vi "Configure RawData.vi"(7 "status?":bool, 8 "error in":errorcluster caption="error in (no error)", 9 "option":i32(ring) items=["ELEM", "SAVE"], 10 "channel":i32(ring) items=["ELEM1", "ELEM2", "ELEM3", "ELEM4", "ELEM5", "ELEM6", "ELEM7"], 11 "VISA resource name":refnum<visa-resource-name>) -> (0 "error out":errorcluster, 3 "VISA resource out":refnum<visa-resource-name>)   [LabVIEW 2018, in "Suita SPAW7000.lvlib"]
uses:
  <instrlib>/Suita SPAW7000/Suita SPAW7000.lvlib
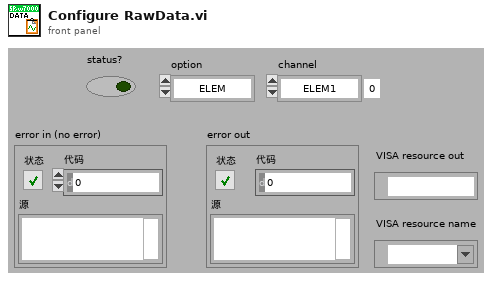
[diagram p1: front panel]
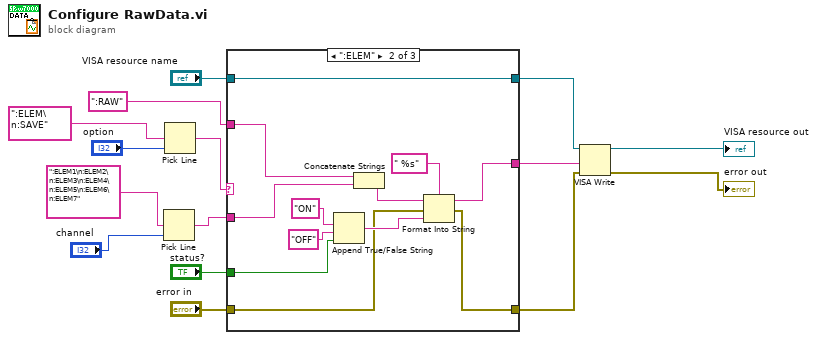
[diagram p0: block diagram]
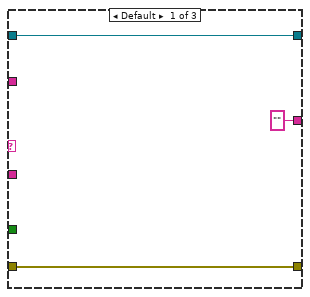
[diagram p2: hidden frame]
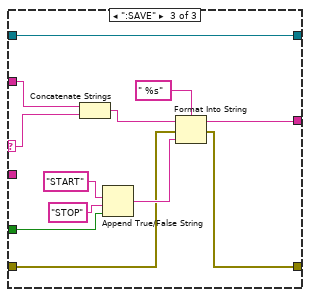
[diagram p3: hidden frame]
diagram:
  n1 = Pick Line(multi-line string=":ELEM1\n:ELEM2\n:ELEM3\n:ELEM4\n:ELEM5\n:ELEM6\n:ELEM7" ("¡s¶ñ"), line index="channel") -> (output string=w12:string)  [unwired: 1 in]
  n2 = Pick Line(multi-line string=":ELEM\n:SAVE" ("¡s¶ñ"), line index="option") -> (output string=w11:string)  [unwired: 1 in]
  n3 = case shown="\":ELEM\"" w11 {
    selector: w11 -> [_ _ w38]
    tunnel: ":RAW" -> [_ w30 w39]
    tunnel: w12 -> [_ w29 _]
    tunnel: "status?" -> [_ w28 w41]
    tunnel: ["" w22 w32] -> w5
    tunnel: "error in" -> [w18 w20 w34]
    tunnel: [w18 w19 w33] -> w3
    tunnel: "VISA resource name" -> [w17 w21 w31]
    tunnel: [w17 w21 w31] -> w1
    frame Default {
    }
    frame ":ELEM" {
      n4 = Append True/False String(1:w28, 2:"OFF" ("假字符串"), 3:"ON" ("真字符串")) -> (0:w25:string)  [unwired: 1 in]
      n5 = Concatenate Strings(w30, w29) -> (w24:string)
      n6 = Format Into String(format string=" %s" ("格式字符串"), initial string=w24, error in=w20, w25) -> (resulting string=w22:string, error out=w19:errorcluster)
    }
    frame ":SAVE" {
      n7 = Concatenate Strings(w39, w38) -> (w36:string)
      n8 = Append True/False String(1:w41, 2:"STOP" ("假字符串"), 3:"START" ("真字符串")) -> (0:w37:string)  [unwired: 1 in]
      n9 = Format Into String(format string=" %s" ("格式字符串"), initial string=w36, error in=w34, w37) -> (resulting string=w32:string, error out=w33:errorcluster)
    }
  }
  n10 = VISA Write(VISA resource name=w1, write buffer=w5, error in (no error)=w3) -> (VISA resource name out=→"VISA resource out":refnum<visa-resource-name>, error out=→"error out":errorcluster)  [unwired: 1 out]
